vi "Err Future Has Expired.vi"() -> (0 "Future Expired":errorcluster)   [LabVIEW 2017, in "Futures.lvlib" / "Future.lvclass"]
uses:
  Future.lvclass
  <vilib>/Utility/error.llb/Error Cluster From Error Code.vi
  <vilib>/ErrorRing/Error Ring.xnode
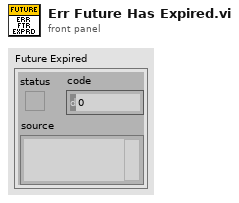
[diagram p1: front panel]
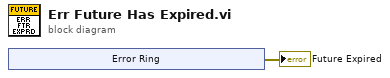
[diagram p0: block diagram]
diagram:
  n1 = xnode "Error Ring"() -> ("error out"=→"Future Expired":errorcluster)
